vi "map_diag.vi"() -> ()   [LabVIEW 2011]
panel:
  in  "OK Button 2":bool
  in  "step (mm)":string
  in  "lato (1=sx,  0 = dx) dal PC":string
  in  "lunghezza da misurare (+ PC, - DOOR)":string
  in  "OK Button":bool
  in  "mm":dbl
  in  "Motor":u16(ring) items=["X", "Y", "Z", "Gluer", "Spint"]
  in  "KILL":bool
  in  "PAUSE":bool
  in  "RESUME":bool
  in  "QUIT":bool
  in  "up done":bool
  in  "z up":bool
  in  "Done":bool
  in  "z piastra 2":bool
  in  "z piastra":bool
  in  "y piastra":bool
  in  "x piastra":bool
  in  "End":bool
  in  "zero z - end":bool
  in  "zero x - end":bool
  in  "zero y - end":bool
  in  "positioning done":bool
  out "output":string
  out "command":string
  in  "zero done":bool
  in  "zero z":bool
  in  "zero x":bool
  in  "zero y":bool
  # "Comandi di emergenza"
  # "Posiziono in zero"
  # "Vado sulla piastra \ne azzero"
  # "Alzo il comparatore"
  # "Vado in posizione"
  # "Ritorno a zero"
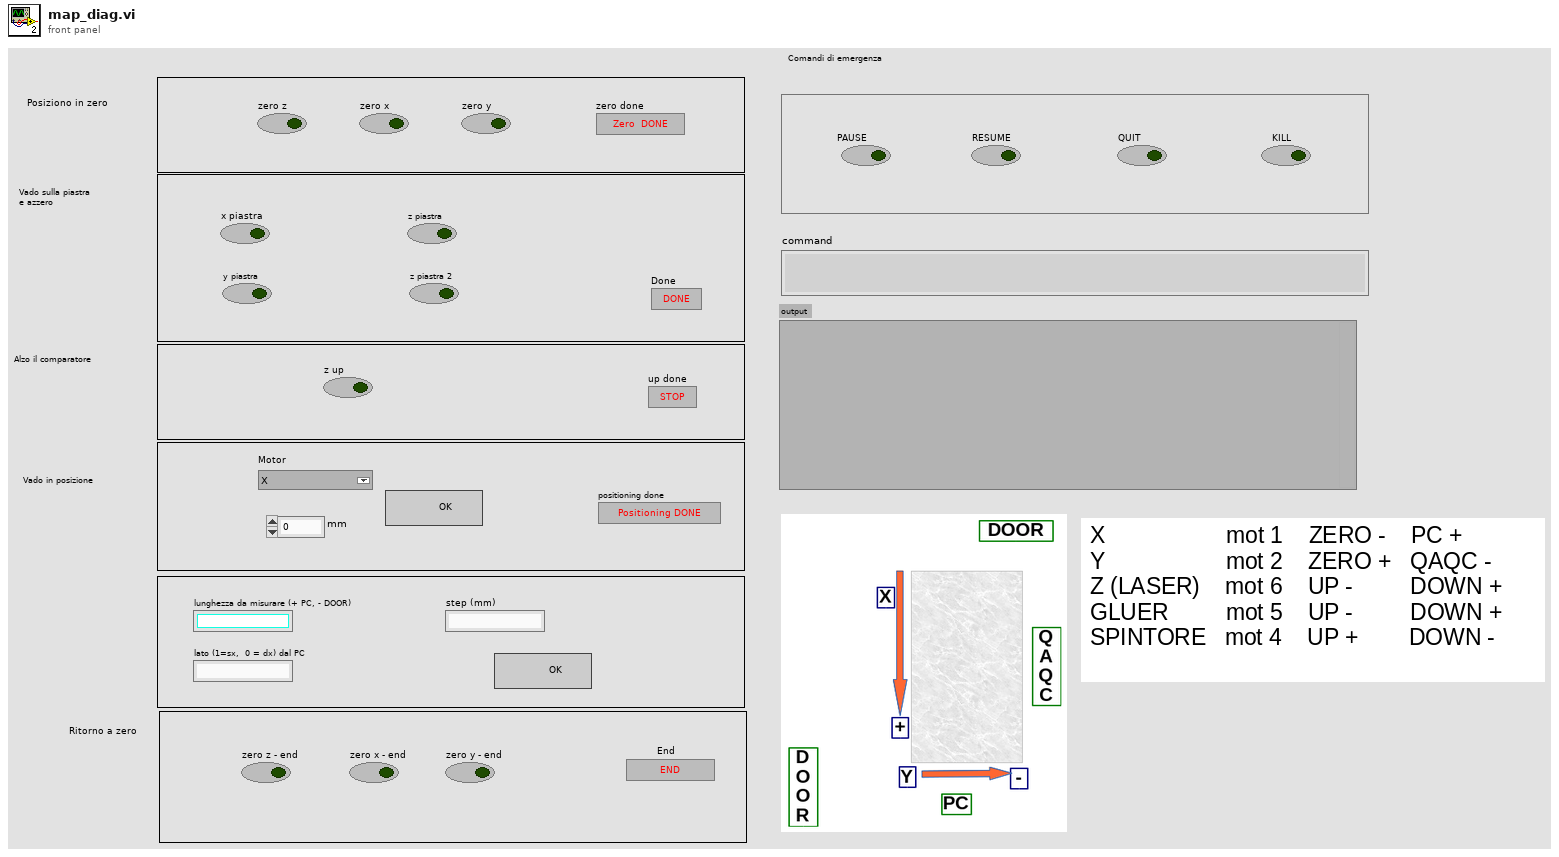
[diagram p1: front panel]
types:
  T1 = enum16{"open", "replace", "create", "open or create", "replace or create", "replace or create with confirmation"}
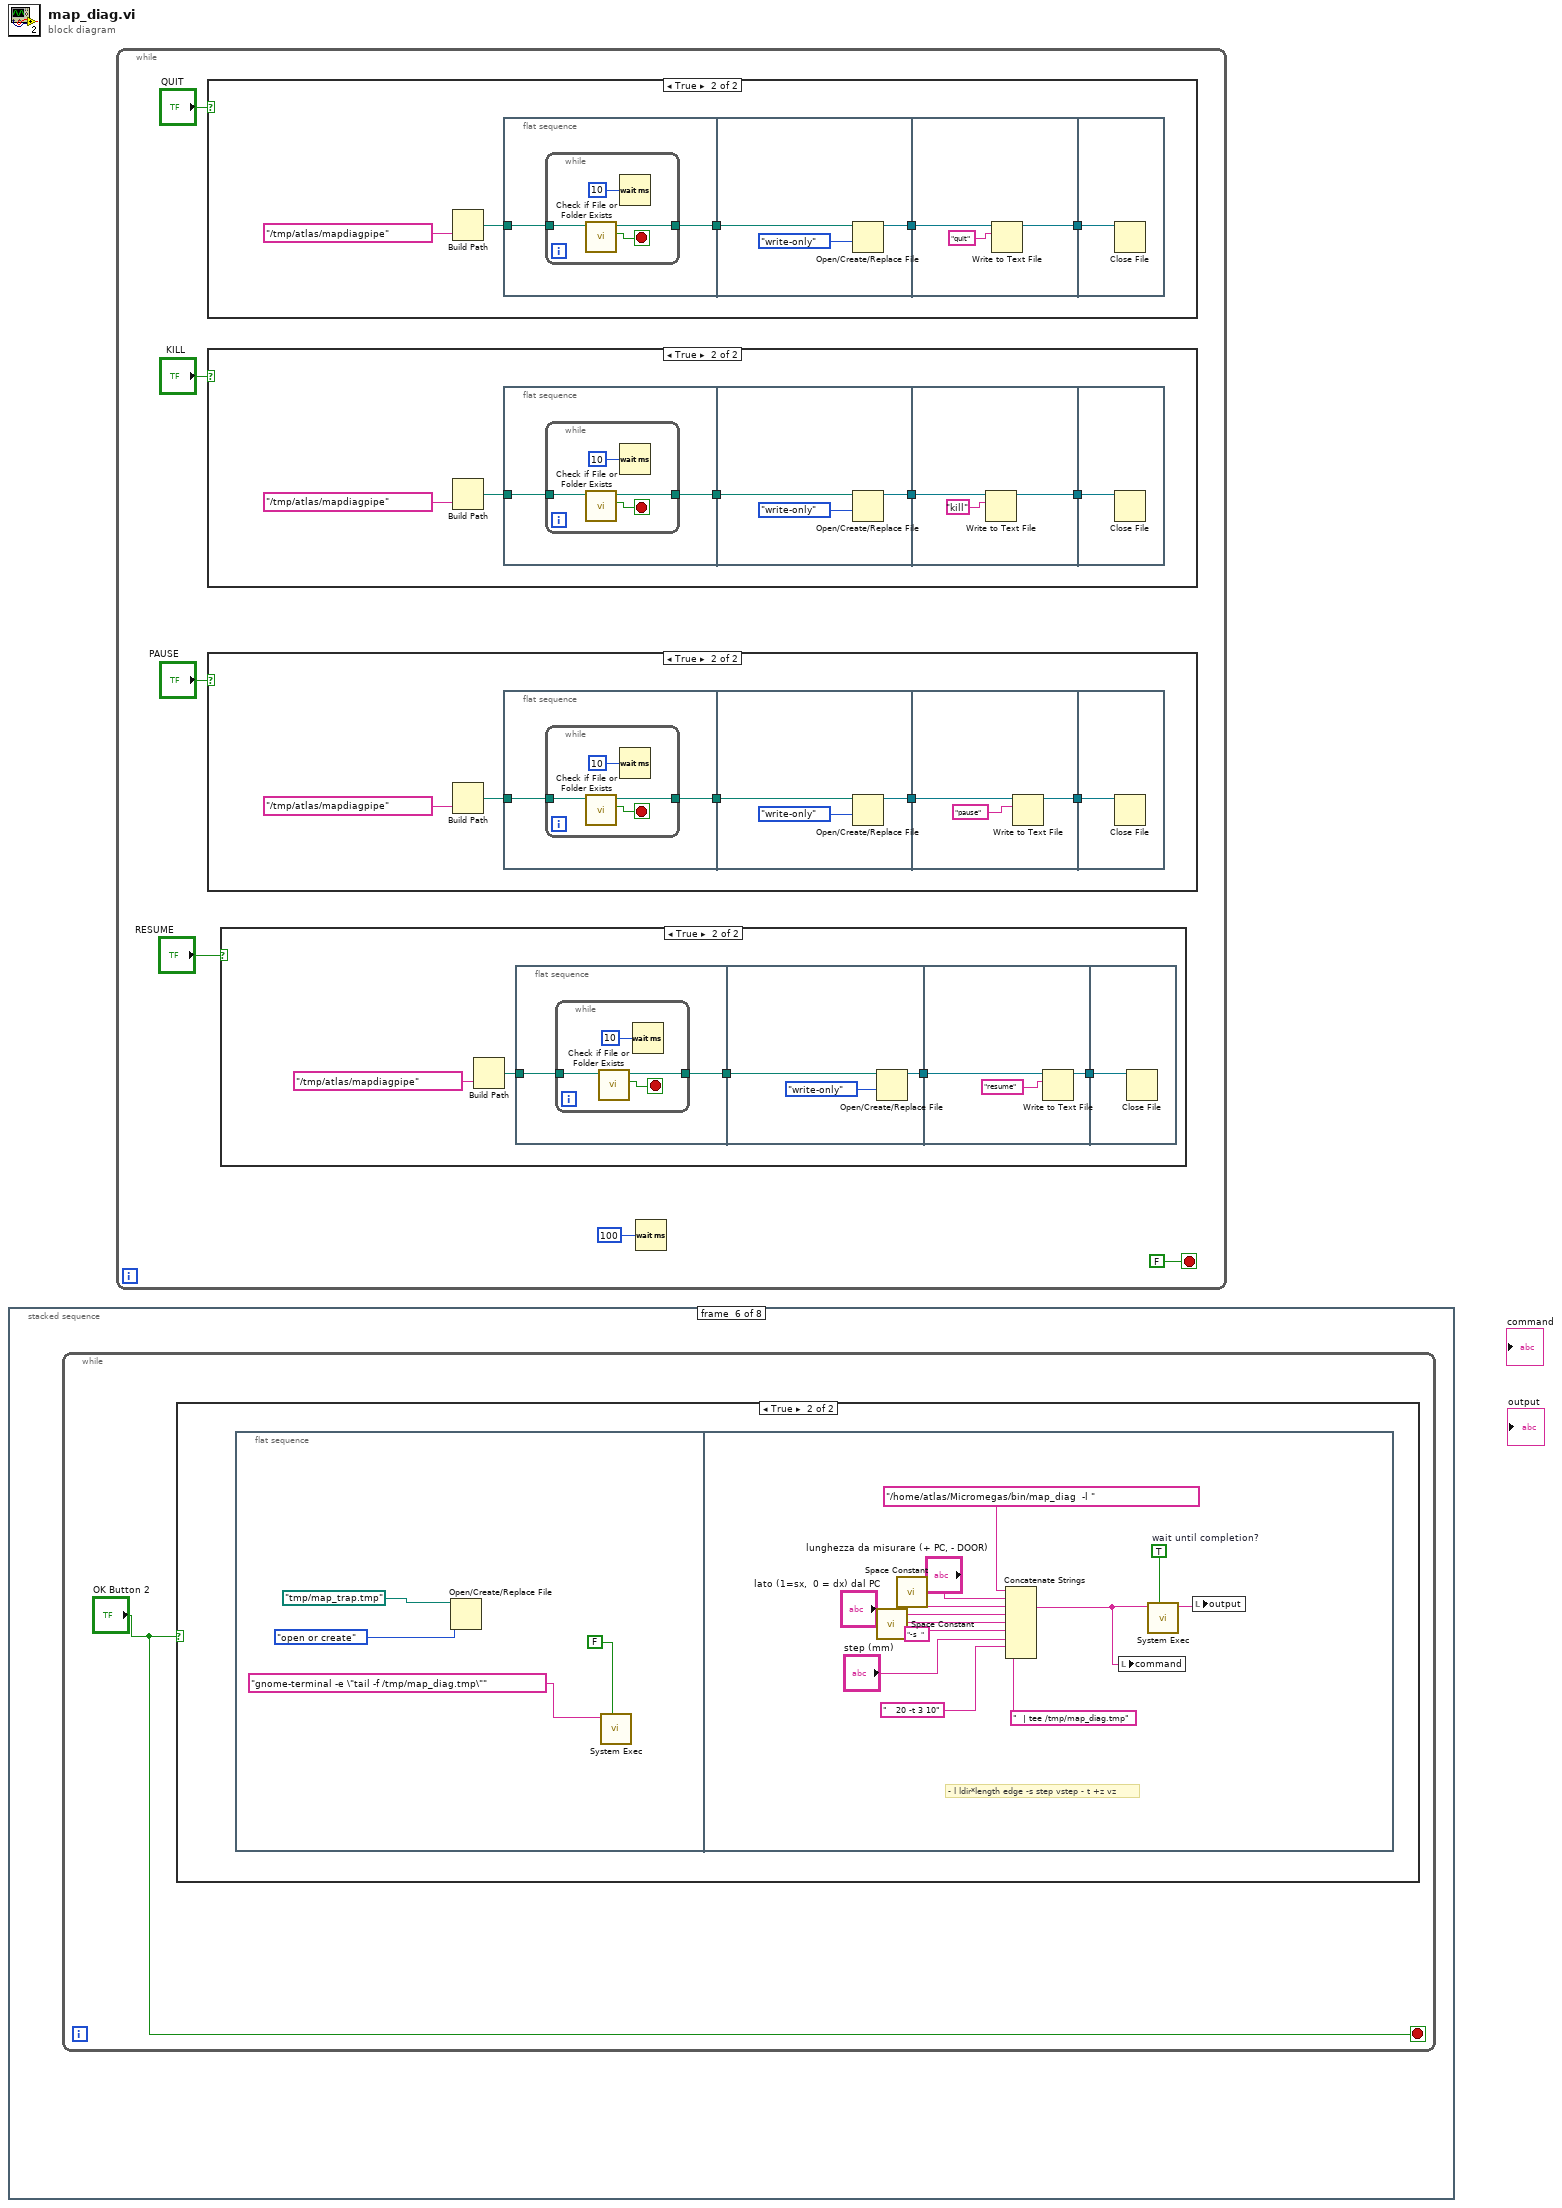
[diagram p0: block diagram]
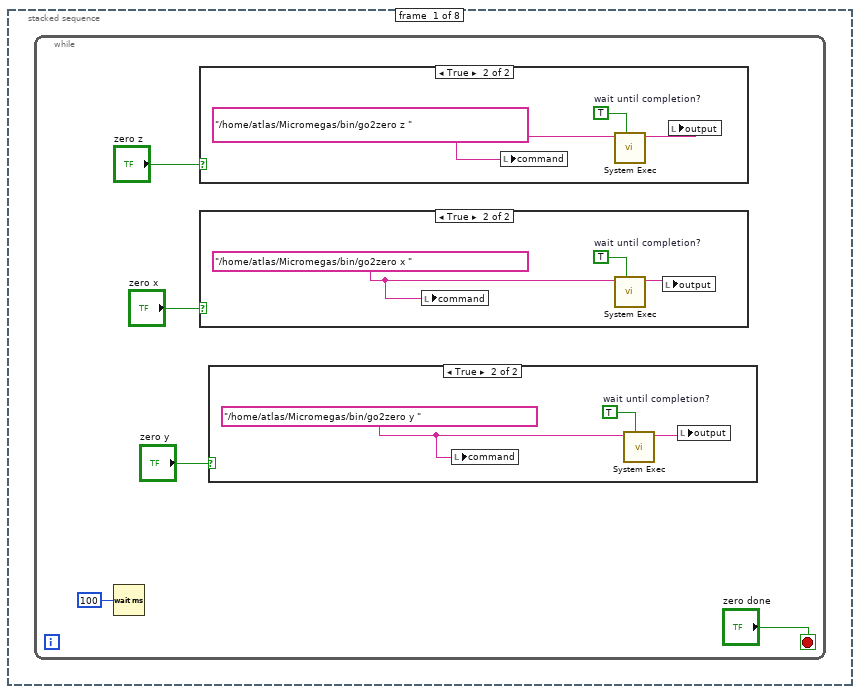
[diagram p6: hidden frame]
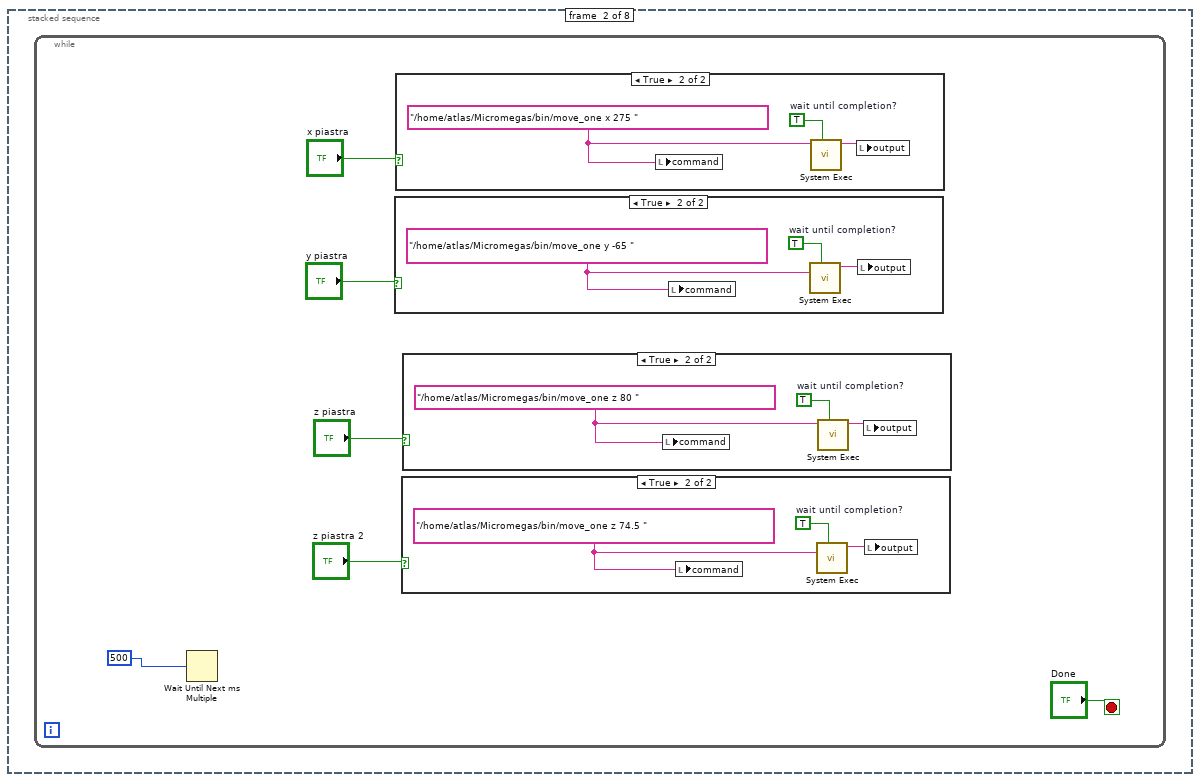
[diagram p10: hidden frame]
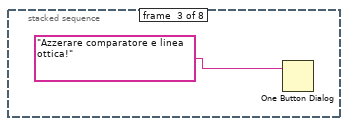
[diagram p15: hidden frame]
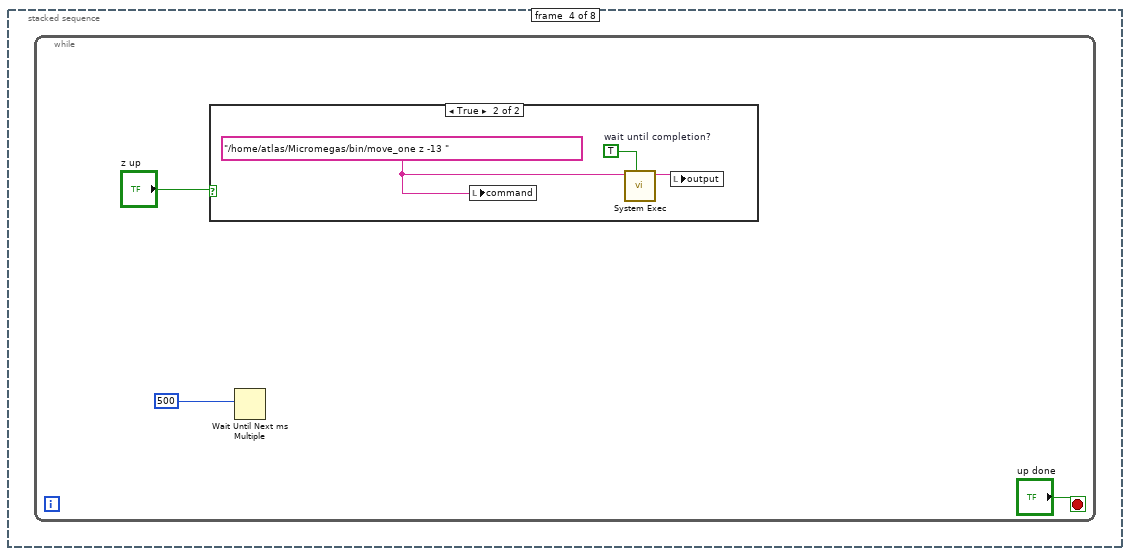
[diagram p16: hidden frame]
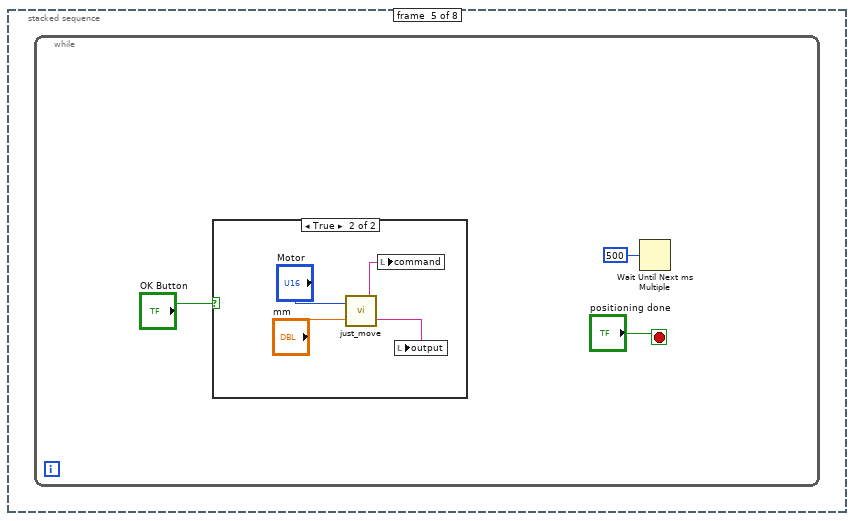
[diagram p18: hidden frame]
diagram:
  n1 = stacked-sequence {
    frame #0 {
      n2 = while {
        stop <- "zero done" stop-if-true
        n3 = Wait (ms)(milliseconds to wait=u32 100) -> ()  [unwired: 1 out]
        n4 = case shown="True" "zero z" {
          frame False {
          }
          frame True {
            w13 = "/home/atlas/Micromegas/bin/go2zero z " ("string")
            w14 = TRUE  # wait until completion?
            n5 = local write "command"(w13) -> ()
            n6 = call <vilib>:"System Exec.vi"("wait until completion? (T)"=w14, "command line"=w13) -> ("standard output"=w12:string)  [unwired: 6 in, 3 out]
            n7 = local write "output"(w12) -> ()
          }
        }
        n8 = case shown="True" "zero x" {
          frame False {
          }
          frame True {
            w10 = "/home/atlas/Micromegas/bin/go2zero x " ("string")
            w11 = TRUE  # wait until completion?
            n9 = local write "command"(w10) -> ()
            n10 = call <vilib>:"System Exec.vi"("wait until completion? (T)"=w11, "command line"=w10) -> ("standard output"=w9:string)  [unwired: 6 in, 3 out]
            n11 = local write "output"(w9) -> ()
          }
        }
        n12 = case shown="True" "zero y" {
          frame False {
          }
          frame True {
            w7 = "/home/atlas/Micromegas/bin/go2zero y " ("string")
            w8 = TRUE  # wait until completion?
            n13 = local write "command"(w7) -> ()
            n14 = call <vilib>:"System Exec.vi"("wait until completion? (T)"=w8, "command line"=w7) -> ("standard output"=w6:string)  [unwired: 6 in, 3 out]
            n15 = local write "output"(w6) -> ()
          }
        }
      }
    }
    frame #1 {
      n16 = while {
        stop <- "Done" stop-if-true
        n17 = Wait Until Next ms Multiple(millisecond multiple=u32 500 ("millisecond timer value")) -> ()  [unwired: 1 out]
        n18 = case shown="True" "y piastra" {
          frame False {
          }
          frame True {
            w27 = "/home/atlas/Micromegas/bin/move_one y -65 " ("string")
            w29 = TRUE  # wait until completion?
            n19 = local write "command"(w27) -> ()
            n20 = call <vilib>:"System Exec.vi"("wait until completion? (T)"=w29, "command line"=w27) -> ("standard output"=w28:string)  [unwired: 6 in, 3 out]
            n21 = local write "output"(w28) -> ()
          }
        }
        n22 = case shown="True" "x piastra" {
          frame False {
          }
          frame True {
            w30 = "/home/atlas/Micromegas/bin/move_one x 275 " ("string")
            w32 = TRUE  # wait until completion?
            n23 = local write "command"(w30) -> ()
            n24 = call <vilib>:"System Exec.vi"("wait until completion? (T)"=w32, "command line"=w30) -> ("standard output"=w31:string)  [unwired: 6 in, 3 out]
            n25 = local write "output"(w31) -> ()
          }
        }
        n26 = case shown="True" "z piastra 2" {
          frame False {
          }
          frame True {
            w21 = "/home/atlas/Micromegas/bin/move_one z 74.5 " ("string")
            w23 = TRUE  # wait until completion?
            n27 = local write "command"(w21) -> ()
            n28 = call <vilib>:"System Exec.vi"("wait until completion? (T)"=w23, "command line"=w21) -> ("standard output"=w22:string)  [unwired: 6 in, 3 out]
            n29 = local write "output"(w22) -> ()
          }
        }
        n30 = case shown="True" "z piastra" {
          frame False {
          }
          frame True {
            w24 = "/home/atlas/Micromegas/bin/move_one z 80 " ("string")
            w26 = TRUE  # wait until completion?
            n31 = local write "command"(w24) -> ()
            n32 = call <vilib>:"System Exec.vi"("wait until completion? (T)"=w26, "command line"=w24) -> ("standard output"=w25:string)  [unwired: 6 in, 3 out]
            n33 = local write "output"(w25) -> ()
          }
        }
      }
    }
    frame #2 {
      n34 = One Button Dialog(message="Azzerare comparatore e linea ottica!") -> ()  [unwired: 1 in, 1 out]
    }
    frame #3 {
      n35 = while {
        stop <- "up done" stop-if-true
        n36 = case shown="True" "z up" {
          frame False {
          }
          frame True {
            w37 = "/home/atlas/Micromegas/bin/move_one z -13 " ("string")
            w39 = TRUE  # wait until completion?
            n37 = local write "command"(w37) -> ()
            n38 = call <vilib>:"System Exec.vi"("wait until completion? (T)"=w39, "command line"=w37) -> ("standard output"=w38:string)  [unwired: 6 in, 3 out]
            n39 = local write "output"(w38) -> ()
          }
        }
        n40 = Wait Until Next ms Multiple(millisecond multiple=u32 500 ("millisecond timer value")) -> ()  [unwired: 1 out]
      }
    }
    frame #4 {
      n41 = while {
        stop <- "positioning done" stop-if-true
        n42 = case shown="True" "OK Button" {
          frame False {
          }
          frame True {
            n43 = call "just_move.vi"("mm"="mm", "Motor"="Motor") -> ("output"=w43:string, "command"=w44:string)
            n44 = local write "command"(w44) -> ()
            n45 = local write "output"(w43) -> ()
          }
        }
        n46 = Wait Until Next ms Multiple(millisecond multiple=u32 500) -> ()  [unwired: 1 out]
      }
    }
    frame #5 {
      n47 = while {
        stop <- "OK Button 2" stop-if-true
        n48 = case shown="True" "OK Button 2" {
          frame False {
          }
          frame True {
            n49 = flat-sequence {
              frame #0 {
                n50 = Open/Create/Replace File(file path (use dialog)=path "/tmp/map_trap.tmp", operation (0:open)=T1."open or create") -> ()  [unwired: 4 in, 3 out]
                n51 = call <vilib>:"System Exec.vi"("wait until completion? (T)"=FALSE, "command line"="gnome-terminal -e \"tail -f /tmp/map_diag.tmp\"") -> ()  [unwired: 6 in, 4 out]
              }
              frame #1 {
                w63 = TRUE  # wait until completion?
                # "- l ldir*length edge -s step vstep - t +z vz"
                n52 = call <vilib>:"Space Constant.vi"() -> ("String"=w57:string)
                n53 = call <vilib>:"Space Constant.vi"() -> ("String"=w59:string)
                n54 = Concatenate Strings("/home/atlas/Micromegas/bin/map_diag  -l " ("string"), "lunghezza da misurare (+ PC, - DOOR)", w59, "lato (1=sx,  0 = dx) dal PC", w57, "-s  " ("string"), "step (mm)", "   20 -t 3 10" ("string"), "  | tee /tmp/map_diag.tmp" ("string")) -> (w52:string)
                n55 = local write "command"(w52) -> ()
                n56 = call <vilib>:"System Exec.vi"("wait until completion? (T)"=w63, "command line"=w52) -> ("standard output"=w61:string)  [unwired: 6 in, 3 out]
                n57 = local write "output"(w61) -> ()
              }
            }
          }
        }
      }
    }
    frame #6 {
      n58 = while {
        stop <- "End" stop-if-true
        n59 = Wait (ms)(milliseconds to wait=u32 100) -> ()  [unwired: 1 out]
        n60 = case shown="True" "zero z - end" {
          frame False {
          }
          frame True {
            w76 = "/home/atlas/Micromegas/bin/go2zero z " ("string")
            w77 = TRUE  # wait until completion?
            n61 = local write "command"(w76) -> ()
            n62 = call <vilib>:"System Exec.vi"("wait until completion? (T)"=w77, "command line"=w76) -> ("standard output"=w75:string)  [unwired: 6 in, 3 out]
            n63 = local write "output"(w75) -> ()
          }
        }
        n64 = case shown="True" "zero x - end" {
          frame False {
          }
          frame True {
            w73 = "/home/atlas/Micromegas/bin/go2zero x " ("string")
            w74 = TRUE  # wait until completion?
            n65 = local write "command"(w73) -> ()
            n66 = call <vilib>:"System Exec.vi"("wait until completion? (T)"=w74, "command line"=w73) -> ("standard output"=w72:string)  [unwired: 6 in, 3 out]
            n67 = local write "output"(w72) -> ()
          }
        }
        n68 = case shown="True" "zero y - end" {
          frame False {
          }
          frame True {
            w70 = "/home/atlas/Micromegas/bin/go2zero y " ("string")
            w71 = TRUE  # wait until completion?
            n69 = local write "command"(w70) -> ()
            n70 = call <vilib>:"System Exec.vi"("wait until completion? (T)"=w71, "command line"=w70) -> ("standard output"=w69:string)  [unwired: 6 in, 3 out]
            n71 = local write "output"(w69) -> ()
          }
        }
      }
    }
    frame #7 {
      n72 = One Button Dialog(message="Per comodita`, rinominare il file (non verra` comunque sovrascritto)") -> ()  [unwired: 1 in, 1 out]
    }
  }
  n73 = while {
    stop <- FALSE stop-if-true
    n74 = case shown="True" "QUIT" {
      frame False {
      }
      frame True {
        n75 = Build Path(name or relative path="/tmp/atlas/mapdiagpipe" ("string")) -> (appended path=w139:path)  [unwired: 1 in]
        n76 = flat-sequence {
          tunnel: [w145] -> w143
          tunnel: w139 -> [w144]
          tunnel: w143 -> [w152]
          tunnel: [w150] -> w142
          tunnel: w142 -> [w155]
          tunnel: [w154] -> w141
          tunnel: w141 -> [w156]
          frame #0 {
            n77 = while {
              tunnel: [w147] -> w145
              tunnel: w144 -> [w146]
              stop <- w148 stop-if-true
              n78 = call <vilib>:"Check if File or Folder Exists.vi"("path"=w146) -> ("file or folder exists?"=w148:bool, "dup path"=w147:path)  [unwired: 8 in, 1 out]
              n79 = Wait (ms)(milliseconds to wait=u32 10) -> ()  [unwired: 1 out]
            }
          }
          frame #1 {
            n80 = Open/Create/Replace File(file path (use dialog)=w152, access (0:read/write)=enum16{"read/write", "read-only", "write-only"}."write-only") -> (refnum out=w150:refnum<file>)  [unwired: 4 in, 2 out]
          }
          frame #2 {
            n81 = Write to Text File(file (use dialog)=w155, text="quit") -> (refnum out=w154:refnum<file>)  [unwired: 2 in, 2 out]
          }
          frame #3 {
            n82 = Close File(refnum=w156) -> ()  [unwired: 1 in, 2 out]
          }
        }
      }
    }
    n83 = case shown="True" "KILL" {
      frame False {
      }
      frame True {
        n84 = Build Path(name or relative path="/tmp/atlas/mapdiagpipe" ("string")) -> (appended path=w103:path)  [unwired: 1 in]
        n85 = flat-sequence {
          tunnel: [w109] -> w107
          tunnel: w103 -> [w108]
          tunnel: w107 -> [w116]
          tunnel: [w114] -> w106
          tunnel: w106 -> [w119]
          tunnel: [w118] -> w105
          tunnel: w105 -> [w120]
          frame #0 {
            n86 = while {
              tunnel: [w111] -> w109
              tunnel: w108 -> [w110]
              stop <- w112 stop-if-true
              n87 = call <vilib>:"Check if File or Folder Exists.vi"("path"=w110) -> ("file or folder exists?"=w112:bool, "dup path"=w111:path)  [unwired: 8 in, 1 out]
              n88 = Wait (ms)(milliseconds to wait=u32 10) -> ()  [unwired: 1 out]
            }
          }
          frame #1 {
            n89 = Open/Create/Replace File(file path (use dialog)=w116, access (0:read/write)=enum16{"read/write", "read-only", "write-only"}."write-only") -> (refnum out=w114:refnum<file>)  [unwired: 4 in, 2 out]
          }
          frame #2 {
            n90 = Write to Text File(file (use dialog)=w119, text="kill") -> (refnum out=w118:refnum<file>)  [unwired: 2 in, 2 out]
          }
          frame #3 {
            n91 = Close File(refnum=w120) -> ()  [unwired: 1 in, 2 out]
          }
        }
      }
    }
    n92 = case shown="True" "PAUSE" {
      frame False {
      }
      frame True {
        n93 = Build Path(name or relative path="/tmp/atlas/mapdiagpipe" ("string")) -> (appended path=w85:path)  [unwired: 1 in]
        n94 = flat-sequence {
          tunnel: [w91] -> w89
          tunnel: w85 -> [w90]
          tunnel: w89 -> [w98]
          tunnel: [w96] -> w88
          tunnel: w88 -> [w101]
          tunnel: [w100] -> w87
          tunnel: w87 -> [w102]
          frame #0 {
            n95 = while {
              tunnel: [w93] -> w91
              tunnel: w90 -> [w92]
              stop <- w94 stop-if-true
              n96 = call <vilib>:"Check if File or Folder Exists.vi"("path"=w92) -> ("file or folder exists?"=w94:bool, "dup path"=w93:path)  [unwired: 8 in, 1 out]
              n97 = Wait (ms)(milliseconds to wait=u32 10) -> ()  [unwired: 1 out]
            }
          }
          frame #1 {
            n98 = Open/Create/Replace File(file path (use dialog)=w98, access (0:read/write)=enum16{"read/write", "read-only", "write-only"}."write-only") -> (refnum out=w96:refnum<file>)  [unwired: 4 in, 2 out]
          }
          frame #2 {
            n99 = Write to Text File(file (use dialog)=w101, text="pause") -> (refnum out=w100:refnum<file>)  [unwired: 2 in, 2 out]
          }
          frame #3 {
            n100 = Close File(refnum=w102) -> ()  [unwired: 1 in, 2 out]
          }
        }
      }
    }
    n101 = case shown="True" "RESUME" {
      frame False {
      }
      frame True {
        n102 = Build Path(name or relative path="/tmp/atlas/mapdiagpipe" ("string")) -> (appended path=w121:path)  [unwired: 1 in]
        n103 = flat-sequence {
          tunnel: [w127] -> w125
          tunnel: w121 -> [w126]
          tunnel: w125 -> [w134]
          tunnel: [w132] -> w124
          tunnel: w124 -> [w137]
          tunnel: [w136] -> w123
          tunnel: w123 -> [w138]
          frame #0 {
            n104 = while {
              tunnel: [w129] -> w127
              tunnel: w126 -> [w128]
              stop <- w130 stop-if-true
              n105 = call <vilib>:"Check if File or Folder Exists.vi"("path"=w128) -> ("file or folder exists?"=w130:bool, "dup path"=w129:path)  [unwired: 8 in, 1 out]
              n106 = Wait (ms)(milliseconds to wait=u32 10) -> ()  [unwired: 1 out]
            }
          }
          frame #1 {
            n107 = Open/Create/Replace File(file path (use dialog)=w134, access (0:read/write)=enum16{"read/write", "read-only", "write-only"}."write-only") -> (refnum out=w132:refnum<file>)  [unwired: 4 in, 2 out]
          }
          frame #2 {
            n108 = Write to Text File(file (use dialog)=w137, text="resume") -> (refnum out=w136:refnum<file>)  [unwired: 2 in, 2 out]
          }
          frame #3 {
            n109 = Close File(refnum=w138) -> ()  [unwired: 1 in, 2 out]
          }
        }
      }
    }
    n110 = Wait (ms)(milliseconds to wait=100) -> ()  [unwired: 1 out]
  }
